vi "to CDATA.vi"(11 "String in":string) -> (3 "CDATA String":string)   [LabVIEW 2010]
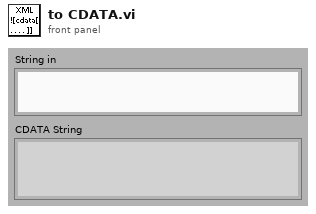
[diagram p1: front panel]
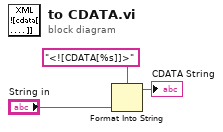
[diagram p0: block diagram]
diagram:
  n1 = Format Into String(format string="<![CDATA[%s]]>", "String in") -> (resulting string=→"CDATA String":string)  [unwired: 2 in, 1 out]
